vi "FR GUI main.vi"() -> ()   [LabVIEW 2020]
doc: "Use this template to build a producer/consumer design pattern with events to produce queue items. Use this design pattern instead of the User Interface Event Hanadler pattern for user interfaces when you want to execute code asynchronously in response to an event without slowing the user interface responsiveness."
uses:
  Type definitions/FRmeter settings.ctl
  General AC source/Type definitions/AC Source.ctl
  General AC source/Type definitions/AC Source type.ctl
  General DC meter/Type definitions/DC meter.ctl
  General DC meter/Type definitions/DC meter type.ctl
  FR Measurement/Type definitions/FR Measuement properties.ctl
  FR Utilities/Type definitions/FR Template definition.ctl
  <vilib>/Utility/error.llb/Error Cluster From Error Code.vi
  <vilib>/ErrorRing/Error Ring.xnode
  external libraries/varilib/varilib.lvlib
panel:
  out "gui_to_hide":refnum<vi>[](array[refnum])
  in  "Skip waiting":bool caption="Abort"
  in  "Setup DCV meter":bool
  out "DC meter status":string caption="DC meter:"
  out "FFmeter settings":T1={"AC Source"={"AC Source type"=enum."Fluke 5XXX calibrator", "VISA"="", "Ref. clock (Hz)"=0.0, "status ref"=refnum}, "TWM pipe"="\\\\.\\pipe\\TWM:server", "Measurement status ref"=refnum, "TWM Status ref"=refnum, "Abort ref"=refnum, "DC meter"={"DC meter type"=enum."H/A/K 3458", "DC meter VISA"="", "NPLC"=10, "status ref"=refnum}, "FR Measurement properties"={"Measurement frequencies (Hz)"=[1000.0], "Sampling frequency (Hz)"=500000.0, "Signal amplitude (V)"=4.5, "AC-DC settle time (s)"=20.0, "Record length (multiples of period)"=[1000.0, 10000.0, 1000.0], "Measurement template file"=path "", "Row of START keyword"=1, "Row of STOP keyword"=0, "Calculate RMS from samples"=FALSE, "AC-DC warm up time (s)"=300.0, "Measurement template line"=[], "DC meter readings No."=10, "Algorithm"="TWM-WFFT", "Simultaneous measurement"=FALSE}, "Skip waiting ref"=refnum, "Octave paths"={"GNU Octave path"=path "C:/Program Files/GNU Octave/Octave-6.2.0/mingw64/bin", "TWM+QWTB path"=path "C:/Users/labina/Desktop/TWM-1.8.7.0-full/octprog", "lvlib path"=path "D:/martin/WAC/WACsw - github/control_software/Filter function meter/external libraries/GOLPI 0.7.3.1 source distribution LV 20.0 32 bit/lv_proc.dll"}, "FR Template definition"={"Keywords column"=0, "Sig. freq. column"=1, "Rec. len. column"=2, "Meas. points. row min to read"=9, "Meas. points. row max to read"=1509, "Properties column"=4, "Properties row start"=1, "Properties row end"=5, "Keyword START regexp"="", "Keyword STOP regexp"="", "HW data column"=7, "HW data row start"=1, "HW data row end"=3, "TIme and date column start"=3, "Digitizer value column start "=4, "DC mean column start "=6, "DC readings column start"=10}, "Recalculate-skip already calculated"=FALSE} {"FR Measurement properties"."Record length (multiples of period)" format="%#_3p"; "FR Measurement properties"."Sampling frequency (Hz)" format="%#_3p"; "FR Measurement properties"."Measurement frequencies (Hz)" format="%#_3p"}
  out "Measurement status:":string
  in  "Setup AC Source":bool
  in  "Measure":bool
  out "gui_unlock_for_measure":refnum<vi>[](array[refnum])
  out "gui_to_lock":refnum<vi>[](array[refnum])
  in  "Setup meas":bool
  in  "Abort":bool
  out "AC source status":string caption="AC source:"
  out "TWM status":string caption="TWM:"
  in  "Setup TWM":bool
  in  "About":bool
  in  "Quit":bool
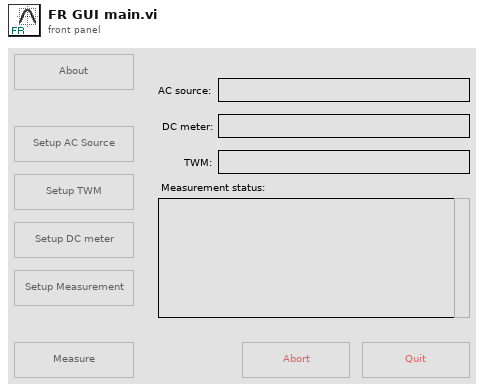
[diagram p1: front panel]
types:
  T1 = typedef "FRmeter settings.ctl" = cluster{"AC Source":T2, "TWM pipe":string, "Measurement status ref":refnum<vi>, "TWM Status ref":refnum<vi>, "Abort ref":refnum<vi>, "DC meter":T4, "FR Measurement properties":T6, "Skip waiting ref":refnum<vi>, "Octave paths":cluster{"GNU Octave path":path, "TWM+QWTB path":path, "lvlib path":path}, "FR Template definition":T7, "Recalculate-skip already calculated":bool}
  T2 = typedef "AC Source.ctl" = cluster{"AC Source type":T3, "VISA":refnum<visa-resource-name>, "Ref. clock (Hz)":dbl, "status ref":refnum<vi>}
  T3 = typedef "AC Source type.ctl" = enum16{"Fluke 5XXX calibrator", "Tektronix AFG3000 series", "dummy"}
  T4 = typedef "DC meter.ctl" = cluster{"DC meter type":T5, "DC meter VISA":refnum<visa-resource-name>, "NPLC":i32, "status ref":refnum<vi>}
  T5 = typedef "DC meter type.ctl" = enum16{"H/A/K 3458", "Fluke 8508A", "dummy", "Keithley 2182"}
  T6 = typedef "FR Measuement properties.ctl" = cluster{"Measurement frequencies (Hz)":dbl[], "Sampling frequency (Hz)":dbl, "Signal amplitude (V)":dbl, "AC-DC settle time (s)":dbl, "Record length (multiples of period)":dbl[], "Measurement template file":path, "Row of START keyword":i32, "Row of STOP keyword":i32, "Calculate RMS from samples":bool, "AC-DC warm up time (s)":dbl, "Measurement template line":i32[], "DC meter readings No.":i32, "Algorithm":string, "Simultaneous measurement":bool}
  T7 = typedef "FR Template definition.ctl" = cluster{"Keywords column":i32, "Sig. freq. column":i32, "Rec. len. column":i32, "Meas. points. row min to read":i32, "Meas. points. row max to read":i32, "Properties column":i32, "Properties row start":i32, "Properties row end":i32, "Keyword START regexp":string, "Keyword STOP regexp":string, "HW data column":i32, "HW data row start":i32, "HW data row end":i32, "TIme and date column start":i32, "Digitizer value column start ":i32, "DC mean column start ":i32, "DC readings column start":i32}
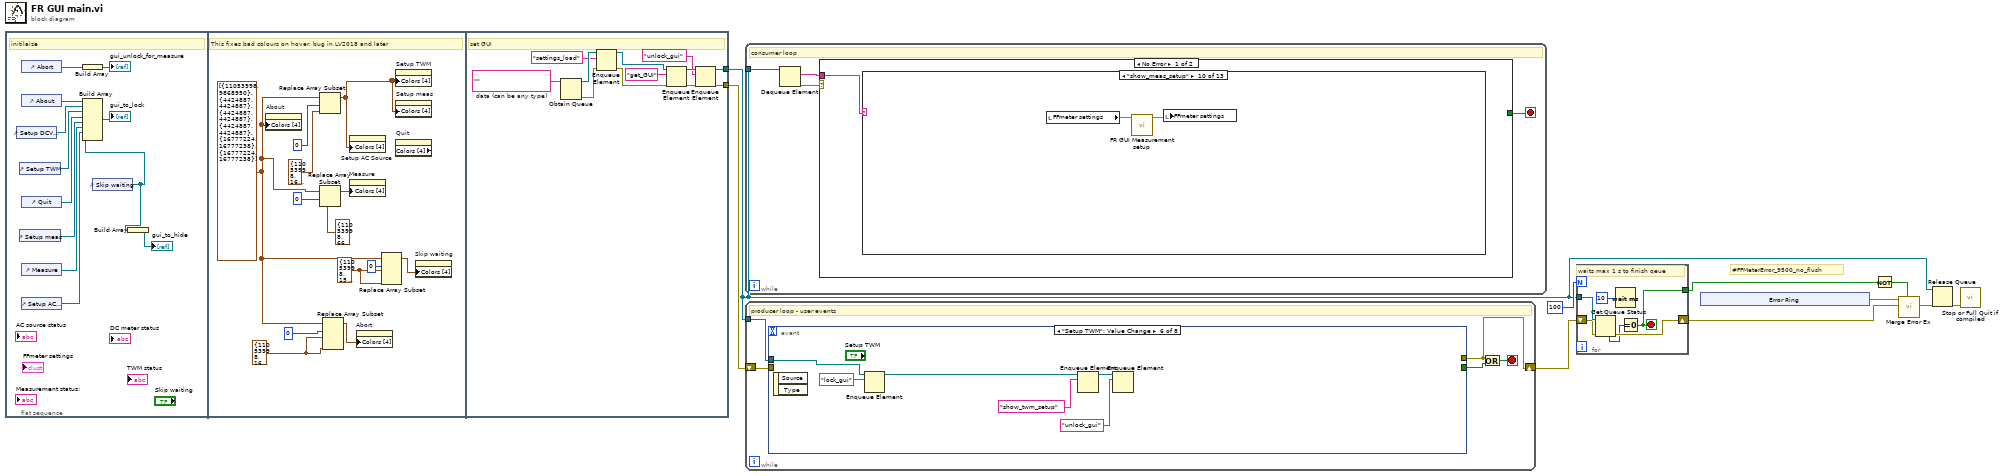
[diagram p0: block diagram]
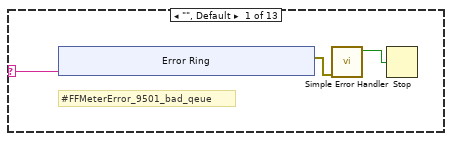
[diagram p2: hidden frame]
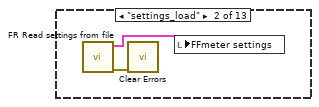
[diagram p3: hidden frame]
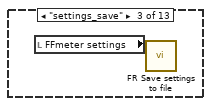
[diagram p4: hidden frame]
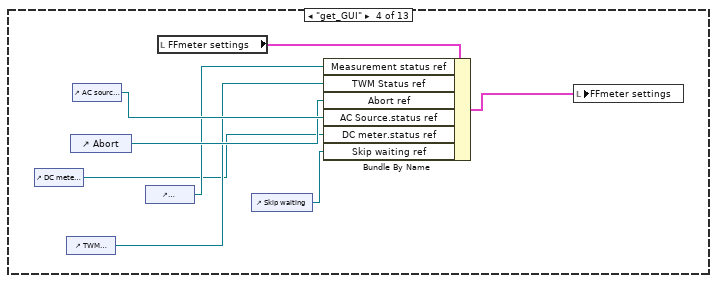
[diagram p5: hidden frame]
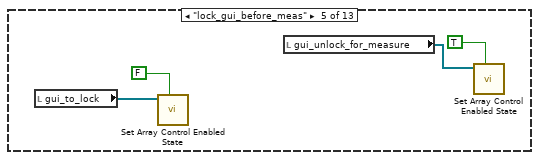
[diagram p6: hidden frame]
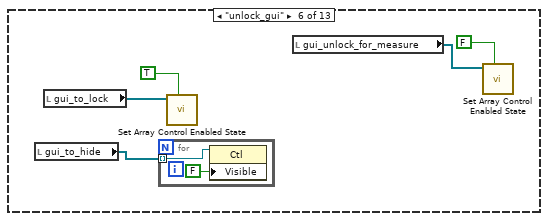
[diagram p7: hidden frame]
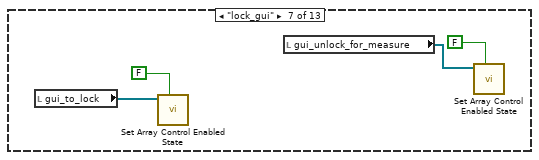
[diagram p8: hidden frame]
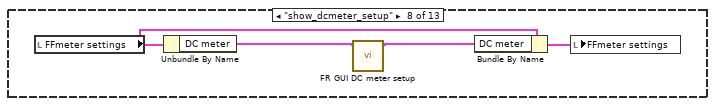
[diagram p9: hidden frame]
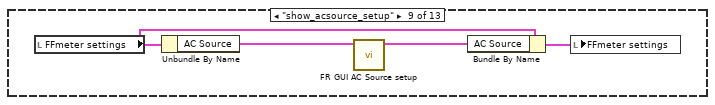
[diagram p10: hidden frame]
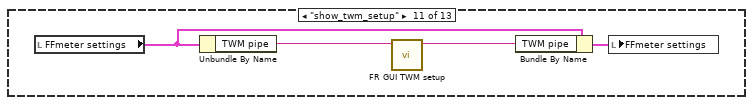
[diagram p11: hidden frame]
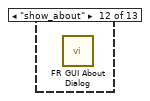
[diagram p12: hidden frame]
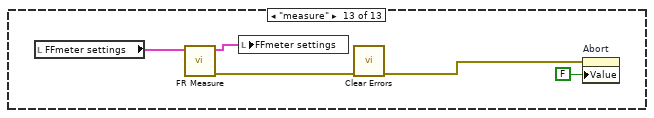
[diagram p13: hidden frame]
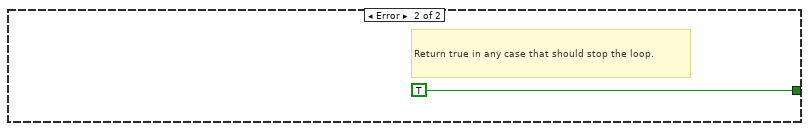
[diagram p14: hidden frame]
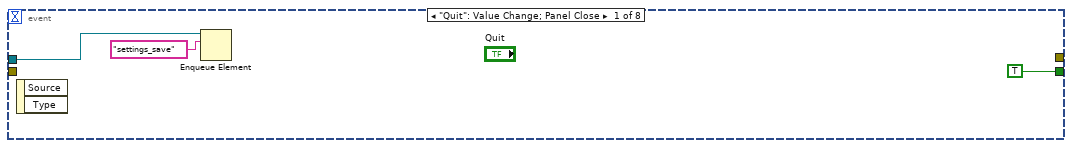
[diagram p15: hidden frame]
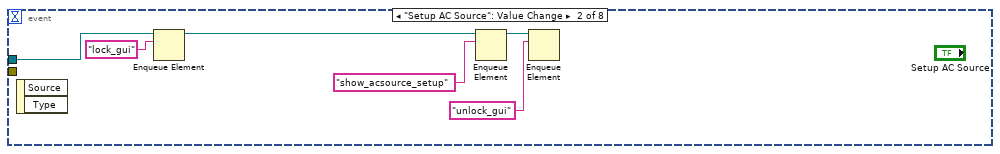
[diagram p16: hidden frame]
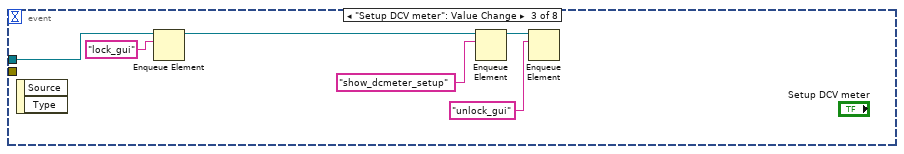
[diagram p17: hidden frame]
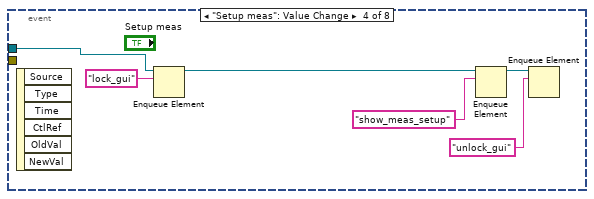
[diagram p18: hidden frame]
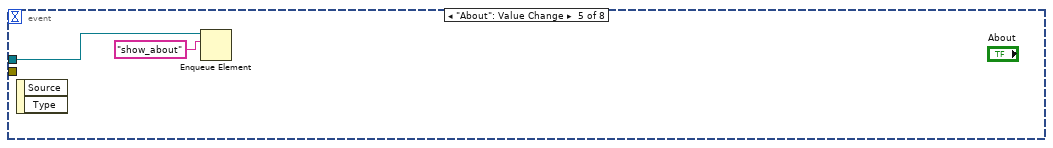
[diagram p19: hidden frame]
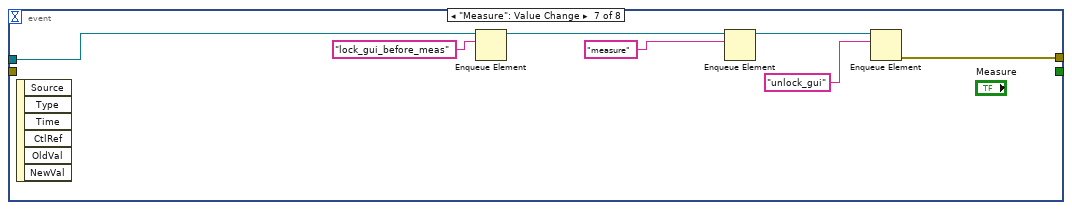
[diagram p20: hidden frame]
diagram:
  # "#FFMeterError_9500_no_flush"
  n1 = flat-sequence {
    tunnel: [w42] -> w4
    tunnel: [w39] -> w10
    frame #0 {
      # "initilaize"
      n2 = control-ref of="Setup DCV meter"() -> (w13:refnum<vi>)
      n3 = control-ref of="Setup TWM"() -> (w17:refnum<vi>)
      n4 = control-ref of="Setup meas"() -> (w19:refnum<vi>)
      n5 = control-ref of="Abort"() -> (w20:refnum<vi>)
      n6 = control-ref of="About"() -> (w16:refnum<vi>)
      n7 = control-ref of="Quit"() -> (w18:refnum<vi>)
      n8 = control-ref of="Measure"() -> (w15:refnum<vi>)
      n9 = control-ref of="Setup AC Source"() -> (w14:refnum<vi>)
      n10 = Build Array(w20) -> (→"gui_unlock_for_measure":refnum<vi>[])
      n11 = control-ref of="Skip waiting"() -> (w12:refnum<vi>)
      n12 = Build Array(w16, w13, w17, w18, w19, w15, w14, w12) -> (→"gui_to_lock":refnum<vi>[])
      n13 = Build Array(w12) -> (→"gui_to_hide":refnum<vi>[])
    }
    frame #1 {
      w24 = cluster{u32, u32} {11053998, 15466424}
      w23 = cluster{u32, u32} {11053998, 16748945}
      w27 = cluster{u32, u32}[] [{11053998, 9868950}, {4424887, 4424887}, {4424887, 4424887}, {4424887, 4424887}, {16777224, 16777238}, {16777224, 16777238}] ("Colors [4]")
      # "This fixes bad colours on hover, bug in LV2018 and later"
      n14 = property on="About" class="Bool"("Colors [4]"=w27) -> ()  [unwired: 2 in, 2 out]
      n15 = Replace Array Subset(array=w27, new element=cluster{u32, u32} {11053998, 16776960}, index=0) -> (w35:cluster{u32, u32}[])
      n16 = Replace Array Subset(array=w27, new element=cluster{u32, u32} {11053998, 6618880}, index=0) -> (w33:cluster{u32, u32}[])
      n17 = Replace Array Subset(array=w27, new element #1=w23, index #1=0 ("index"), new element #2=w23) -> (w34:cluster{u32, u32}[])  [unwired: 1 in]
      n18 = property on="Setup AC Source" class="Bool"("Colors [4]"=w35) -> ()  [unwired: 2 in, 2 out]
      n19 = property on="Measure" class="Bool"("Colors [4]"=w33) -> ()  [unwired: 2 in, 2 out]
      n20 = property on="Abort" class="Bool (strict)"("Colors [4]"=w34) -> ()  [unwired: 2 in, 2 out]
      n21 = Replace Array Subset(array=w27, new element #1=w24, index #1=0 ("index"), new element #2=w24) -> (w26:cluster{u32, u32}[])  [unwired: 1 in]
      n22 = property on="Setup TWM" class="Bool"("Colors [4]"=w35) -> ()  [unwired: 2 in, 2 out]
      n23 = property on="Setup meas" class="Bool"("Colors [4]"=w35) -> ()  [unwired: 2 in, 2 out]
      n24 = property on="Quit" class="Bool" props=["Colors [4]"]() -> ()  [unwired: 2 in, 3 out]
      n25 = property on="Skip waiting" class="Bool (strict)"("Colors [4]"=w26) -> ()  [unwired: 2 in, 2 out]
    }
    frame #2 {
      w47 = ""  # data (can be any type)
      # "set GUI"
      n26 = Obtain Queue(element data type=w47) -> (queue out=w46:refnum<queue>, error out=w45:errorcluster)  [unwired: 4 in, 1 out]
      n27 = Enqueue Element(queue=w46, element="settings_load", error in (no error)=w45) -> (queue out=w37:refnum<queue>, error out=w36:errorcluster)  [unwired: 1 in, 1 out]
      n28 = Enqueue Element(queue=w37, element="get_GUI", error in (no error)=w36) -> (queue out=w40:refnum<queue>, error out=w41:errorcluster)  [unwired: 1 in, 1 out]
      n29 = Enqueue Element(queue=w40, element="unlock_gui", error in (no error)=w41) -> (queue out=w42:refnum<queue>, error out=w39:errorcluster)  [unwired: 1 in, 1 out]
    }
  }
  n30 = while {
    tunnel: w4 -> [w51]
    stop <- w48 stop-if-true
    # "consumer loop"
    n31 = Dequeue Element(queue=w51) -> (element=w49:string, error out=w50:errorcluster)  [unwired: 2 in, 2 out]
    n32 = case shown="No Error" w50 {
      tunnel: w49 -> [w52 _]
      tunnel: [_ TRUE] -> w48
      frame No Error {
        n33 = case shown="\"show_meas_setup\"" w52 {
          selector: w52 -> [w53 _ _ _ _ _ _ _ _ _ _ _ _]
          frame "", Default {
            # "#FFMeterError_9501_bad_qeue"
            n34 = xnode "Error Ring"("parameter 0"=w53) -> ("error out"=w55:errorcluster)
            n35 = call <vilib>:"Simple Error Handler.vi"("error in (no error)"=w55) -> ("error?"=w54:bool)  [unwired: 4 in, 4 out]
            n36 = Stop(stop? (T)=w54) -> ()
          }
          frame "settings_load" {
            n37 = call "FR Read settings from file.vi"() -> ("error out"=w63:errorcluster, "FFmeter settings"=w64:T1)  [unwired: 10 in]
            n38 = call <vilib>:"Clear Errors.vi"("error in (no error)"=w63) -> ()  [unwired: 5 in, 2 out]
            n39 = local write "FFmeter settings"(w64) -> ()
          }
          frame "settings_save" {
            n40 = local read "FFmeter settings"() -> (w65:T1)
            n41 = call "FR Save settings to file.vi"("FFmeter settings"=w65) -> ()  [unwired: 10 in, 1 out]
          }
          frame "get_GUI" {
            n42 = control-ref of="DC meter status"() -> (w67:refnum<vi>)
            n43 = control-ref of="TWM status"() -> (w68:refnum<vi>)
            n44 = control-ref of="Abort"() -> (w70:refnum<vi>)
            n45 = control-ref of="AC source status"() -> (w71:refnum<vi>)
            n46 = control-ref of="Measurement status:"() -> (w69:refnum<vi>)
            n47 = local read "FFmeter settings"() -> (w73:T1)
            n48 = control-ref of="Skip waiting"() -> (w66:refnum<vi>)
            n49 = Bundle By Name(cluster=w73, "Measurement status ref"=w69, "TWM Status ref"=w68, "Abort ref"=w70, "AC Source.status ref"=w71, "DC meter.status ref"=w67, "Skip waiting ref"=w66) -> (w72:T1)
            n50 = local write "FFmeter settings"(w72) -> ()
          }
          frame "lock_gui_before_meas" {
            n51 = local read "gui_to_lock"() -> (w77:refnum<vi>[])
            n52 = call "Set Array Control Enabled State.vi"("enabled (T)"=FALSE, "reference array in"=w77) -> ()  [unwired: 8 in, 2 out]
            n53 = local read "gui_unlock_for_measure"() -> (w75:refnum<vi>[])
            n54 = call "Set Array Control Enabled State.vi"("enabled (T)"=TRUE, "reference array in"=w75) -> ()  [unwired: 8 in, 2 out]
          }
          frame "unlock_gui" {
            n55 = local read "gui_to_hide"() -> (w78:refnum<vi>[])
            n56 = local read "gui_to_lock"() -> (w82:refnum<vi>[])
            n57 = for {
              tunnel: w78 -> [w84] mode=indexing
              n58 = property class="Ctl"(reference=w84, "Visible"=FALSE) -> ()  [unwired: 1 in, 2 out]
            }
            n59 = call "Set Array Control Enabled State.vi"("enabled (T)"=TRUE, "reference array in"=w82) -> ()  [unwired: 8 in, 2 out]
            n60 = local read "gui_unlock_for_measure"() -> (w81:refnum<vi>[])
            n61 = call "Set Array Control Enabled State.vi"("enabled (T)"=FALSE, "reference array in"=w81) -> ()  [unwired: 8 in, 2 out]
          }
          frame "lock_gui" {
            n62 = local read "gui_to_lock"() -> (w88:refnum<vi>[])
            n63 = call "Set Array Control Enabled State.vi"("enabled (T)"=FALSE, "reference array in"=w88) -> ()  [unwired: 8 in, 2 out]
            n64 = local read "gui_unlock_for_measure"() -> (w87:refnum<vi>[])
            n65 = call "Set Array Control Enabled State.vi"("enabled (T)"=FALSE, "reference array in"=w87) -> ()  [unwired: 8 in, 2 out]
          }
          frame "show_dcmeter_setup" {
            n66 = local read "FFmeter settings"() -> (w92:T1)
            n67 = Unbundle By Name(w92) -> ("DC meter"=w90:T4)
            n68 = call "FR GUI DC meter setup.vi"("DC meter"=w90) -> ("DC meter out"=w89:T4)  [unwired: 10 in]
            n69 = Bundle By Name(cluster=w92, "DC meter"=w89) -> (w91:T1)
            n70 = local write "FFmeter settings"(w91) -> ()
          }
          frame "show_acsource_setup" {
            n71 = local read "FFmeter settings"() -> (w96:T1)
            n72 = Unbundle By Name(w96) -> ("AC Source"=w94:T2)
            n73 = call "FR GUI AC Source setup.vi"("AC Source"=w94) -> ("AC Source out"=w93:T2)  [unwired: 10 in]
            n74 = Bundle By Name(cluster=w96, "AC Source"=w93) -> (w95:T1)
            n75 = local write "FFmeter settings"(w95) -> ()
          }
          frame "show_meas_setup" {
            n76 = local read "FFmeter settings"() -> (w98:T1)
            n77 = call "FR GUI Measurement setup.vi"("FFmeter settings"=w98) -> ("FFmeter settings out"=w97:T1)  [unwired: 8 in]
            n78 = local write "FFmeter settings"(w97) -> ()
          }
          frame "show_twm_setup" {
            n79 = local read "FFmeter settings"() -> (w102:T1)
            n80 = Unbundle By Name(w102) -> ("TWM pipe"=w100:string)
            n81 = call "FR GUI TWM setup.vi"("TWM pipe"=w100) -> ("TWM pipe out"=w99:string)  [unwired: 10 in]
            n82 = Bundle By Name(cluster=w102, "TWM pipe"=w99) -> (w101:T1)
            n83 = local write "FFmeter settings"(w101) -> ()
          }
          frame "show_about" {
            n84 = call "FR GUI About Dialog.vi"() -> ()  [unwired: 12 in]
          }
          frame "measure" {
            n85 = local read "FFmeter settings"() -> (w107:T1)
            n86 = call "FR Measure.vi"("FFmeter settings"=w107) -> ("error out"=w106:errorcluster, "FFmeter settings out"=w103:T1)  [unwired: 9 in]
            n87 = local write "FFmeter settings"(w103) -> ()
            n88 = call <vilib>:"Clear Errors.vi"("error in (no error)"=w106) -> ("error out"=w105:errorcluster)  [unwired: 5 in, 1 out]
            n89 = property on="Abort" class="Bool (strict)"(error in=w105, "Value"=FALSE ("Abort")) -> ()  [unwired: 1 in, 2 out]
          }
        }
      }
      frame Error {
        # "Return true in any case that should stop the loop."
      }
    }
  }
  n90 = while {
    shift-right: [w109] -> w3
    shift-left: w10 -> [w112]
    tunnel: w4 -> [w113]
    stop <- w110 stop-if-true
    # "producer loop - user events"
    n91 = event shown="[5] \"Setup TWM\": Value Change" {
      selector: _ -> [_ _ _ _ _ _ _ _]
      dyn-events: _ -> [_ _ _ _ _ _ _ _]
      timeout: _ -> [_ _ _ _ _ _ _ _]
      tunnel: w113 -> [w114 w119 w125 w131 w135 w139 w148 _]
      tunnel: w112 -> [_ _ _ _ _ _ _ _]
      tunnel: [_ _ _ _ _ _ w143 _] -> w109
      tunnel: [TRUE ("cancel") _ _ _ _ _ _ _] -> w111
      event "Quit": Value Change; Panel Close {
        n92 = event-data() -> ()  [unwired: 1 in, 2 out]
        n93 = Enqueue Element(queue=w114, element="settings_save") -> ()  [unwired: 2 in, 3 out]
      }
      event "Setup AC Source": Value Change {
        n94 = event-data() -> ()  [unwired: 1 in, 2 out]
        n95 = Enqueue Element(queue=w119, element="lock_gui") -> (queue out=w118:refnum<queue>)  [unwired: 2 in, 2 out]
        n96 = Enqueue Element(queue=w118, element="show_acsource_setup") -> (queue out=w117:refnum<queue>)  [unwired: 2 in, 2 out]
        n97 = Enqueue Element(queue=w117, element="unlock_gui") -> ()  [unwired: 2 in, 3 out]
      }
      event "Setup DCV meter": Value Change {
        n98 = event-data() -> ()  [unwired: 1 in, 2 out]
        n99 = Enqueue Element(queue=w125, element="lock_gui") -> (queue out=w124:refnum<queue>)  [unwired: 2 in, 2 out]
        n100 = Enqueue Element(queue=w124, element="show_dcmeter_setup") -> (queue out=w123:refnum<queue>)  [unwired: 2 in, 2 out]
        n101 = Enqueue Element(queue=w123, element="unlock_gui") -> ()  [unwired: 2 in, 3 out]
      }
      event "Setup meas": Value Change {
        n102 = event-data() -> ()  [unwired: 1 in, 6 out]
        n103 = Enqueue Element(queue=w131, element="lock_gui") -> (queue out=w130:refnum<queue>)  [unwired: 2 in, 2 out]
        n104 = Enqueue Element(queue=w130, element="show_meas_setup") -> (queue out=w129:refnum<queue>)  [unwired: 2 in, 2 out]
        n105 = Enqueue Element(queue=w129, element="unlock_gui") -> ()  [unwired: 2 in, 3 out]
      }
      event "About": Value Change {
        n106 = event-data() -> ()  [unwired: 1 in, 2 out]
        n107 = Enqueue Element(queue=w135, element="show_about") -> ()  [unwired: 2 in, 3 out]
      }
      event "Setup TWM": Value Change {
        n108 = event-data() -> ()  [unwired: 1 in, 2 out]
        n109 = Enqueue Element(queue=w139, element="lock_gui") -> (queue out=w138:refnum<queue>)  [unwired: 2 in, 2 out]
        n110 = Enqueue Element(queue=w138, element="show_twm_setup") -> (queue out=w137:refnum<queue>)  [unwired: 2 in, 2 out]
        n111 = Enqueue Element(queue=w137, element="unlock_gui") -> ()  [unwired: 2 in, 3 out]
      }
      event "Measure": Value Change {
        n112 = event-data() -> ()  [unwired: 1 in, 6 out]
        n113 = Enqueue Element(queue=w148, element="lock_gui_before_meas") -> (queue out=w147:refnum<queue>)  [unwired: 2 in, 2 out]
        n114 = Enqueue Element(queue=w147, element="measure") -> (queue out=w146:refnum<queue>)  [unwired: 2 in, 2 out]
        n115 = Enqueue Element(queue=w146, element="unlock_gui") -> (error out=w143:errorcluster)  [unwired: 2 in, 2 out]
      }
      event "Abort": Value Change {
        n116 = event-data() -> ()  [unwired: 1 in, 6 out]
        n117 = control-ref of="Abort"() -> (w151:refnum<vi>)
        n118 = call "Set Control Enabled State.vi"("enabled (T)"=FALSE, "reference in"=w151) -> ()  [unwired: 8 in, 2 out]
      }
    }
    n119 = Or(x=w109, y=w111) -> (x .or. y?=w110:bool)
  }
  n120 = for {
    N: 100 -> [_]
    tunnel: w4 -> [w157]
    shift-right: [w155] -> w8
    shift-left: w3 -> [w156]
    tunnel: [w152] -> w6
    stop <- w152 stop-if-true
    # "waits max 1 s to finish qeue"
    n121 = Get Queue Status(queue=w157, error in (no error)=w156) -> (error out=w155:errorcluster, # elements in queue=w153:i32)  [unwired: 1 in, 6 out]
    n122 = Wait (ms)(milliseconds to wait=u32 10) -> ()  [unwired: 1 out]
    n123 = Equal To 0?(x=w153) -> (x = 0?=w152:bool)
  }
  n124 = xnode "Error Ring"() -> ("error out"=w9:errorcluster)
  n125 = Not(x=w6) -> (.not. x?=w7:bool)
  n126 = call "Merge Error Ex.vi"("Is error? (False)"=w7, "main error in (no error)"=w8, "second error in"=w9) -> ("error out"=w2:errorcluster)  [unwired: 8 in]
  n127 = Release Queue(queue=w4, error in (no error)=w2) -> (error out=w1:errorcluster)  [unwired: 1 in, 2 out]
  n128 = call "Stop or Full Quit if compiled.vi"("error in (no effect)"=w1) -> ()  [unwired: 3 in]
